vi "HW_Poll_Tracker_2.0.4+.vi"(8 "error in":errorcluster, 11 "VISA resource name in":refnum<visa-resource-name>="ASRL3::INSTR") -> (0 "error out":errorcluster, 1 "Read buffer":string, 2 "Parameters output":T1, 3 "VISA resource name out":refnum<visa-resource-name>, 4 "Sync mode status":string, 5 "Sensor board size":string)   [LabVIEW 2016]
panel:
  out "Sync mode index":i32
  out "Sensor board index":i32
  out "Sensors response":string
  out "Port data status":i32
  out "Port data status index":i32
  out "FPS status":i32
  out "Poll records":u32
  out "FPS target index":i32
  out "Matrix mode status":string
  out "Matrix mode index":i32
  out "Coordinate mode status":string
  out "Coordinate mode index":i32
  out "Binary mode status":string
  out "Binary mode index":i32
  out "Array of tokens":string[](array[string])
  out "token index":i32
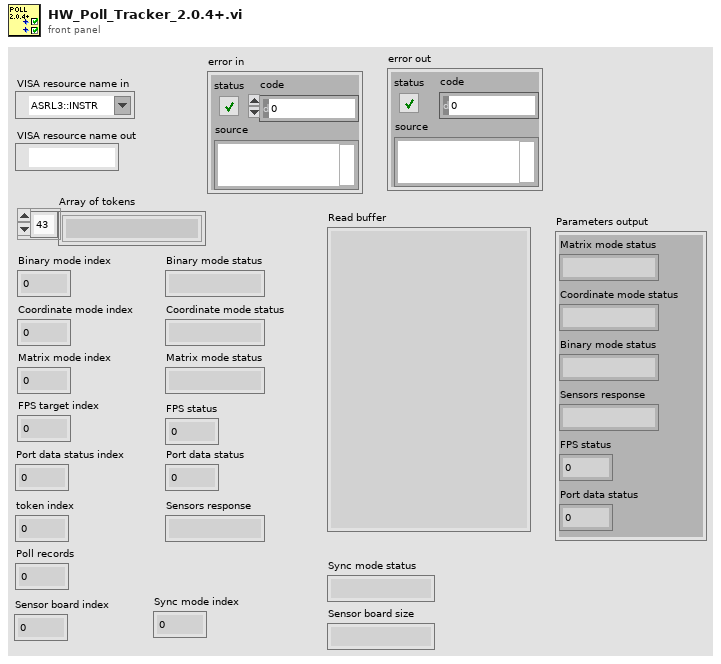
[diagram p1: front panel]
types:
  T1 = cluster{"Matrix mode status":string, "Coordinate mode status":string, "Binary mode status":string, "Sensors response":string, "FPS status":i32, "Port data status":i32}
  T2 = cluster{"token string":string, "token string":string, "token string":string, "trimmed string":string, i32, i32}
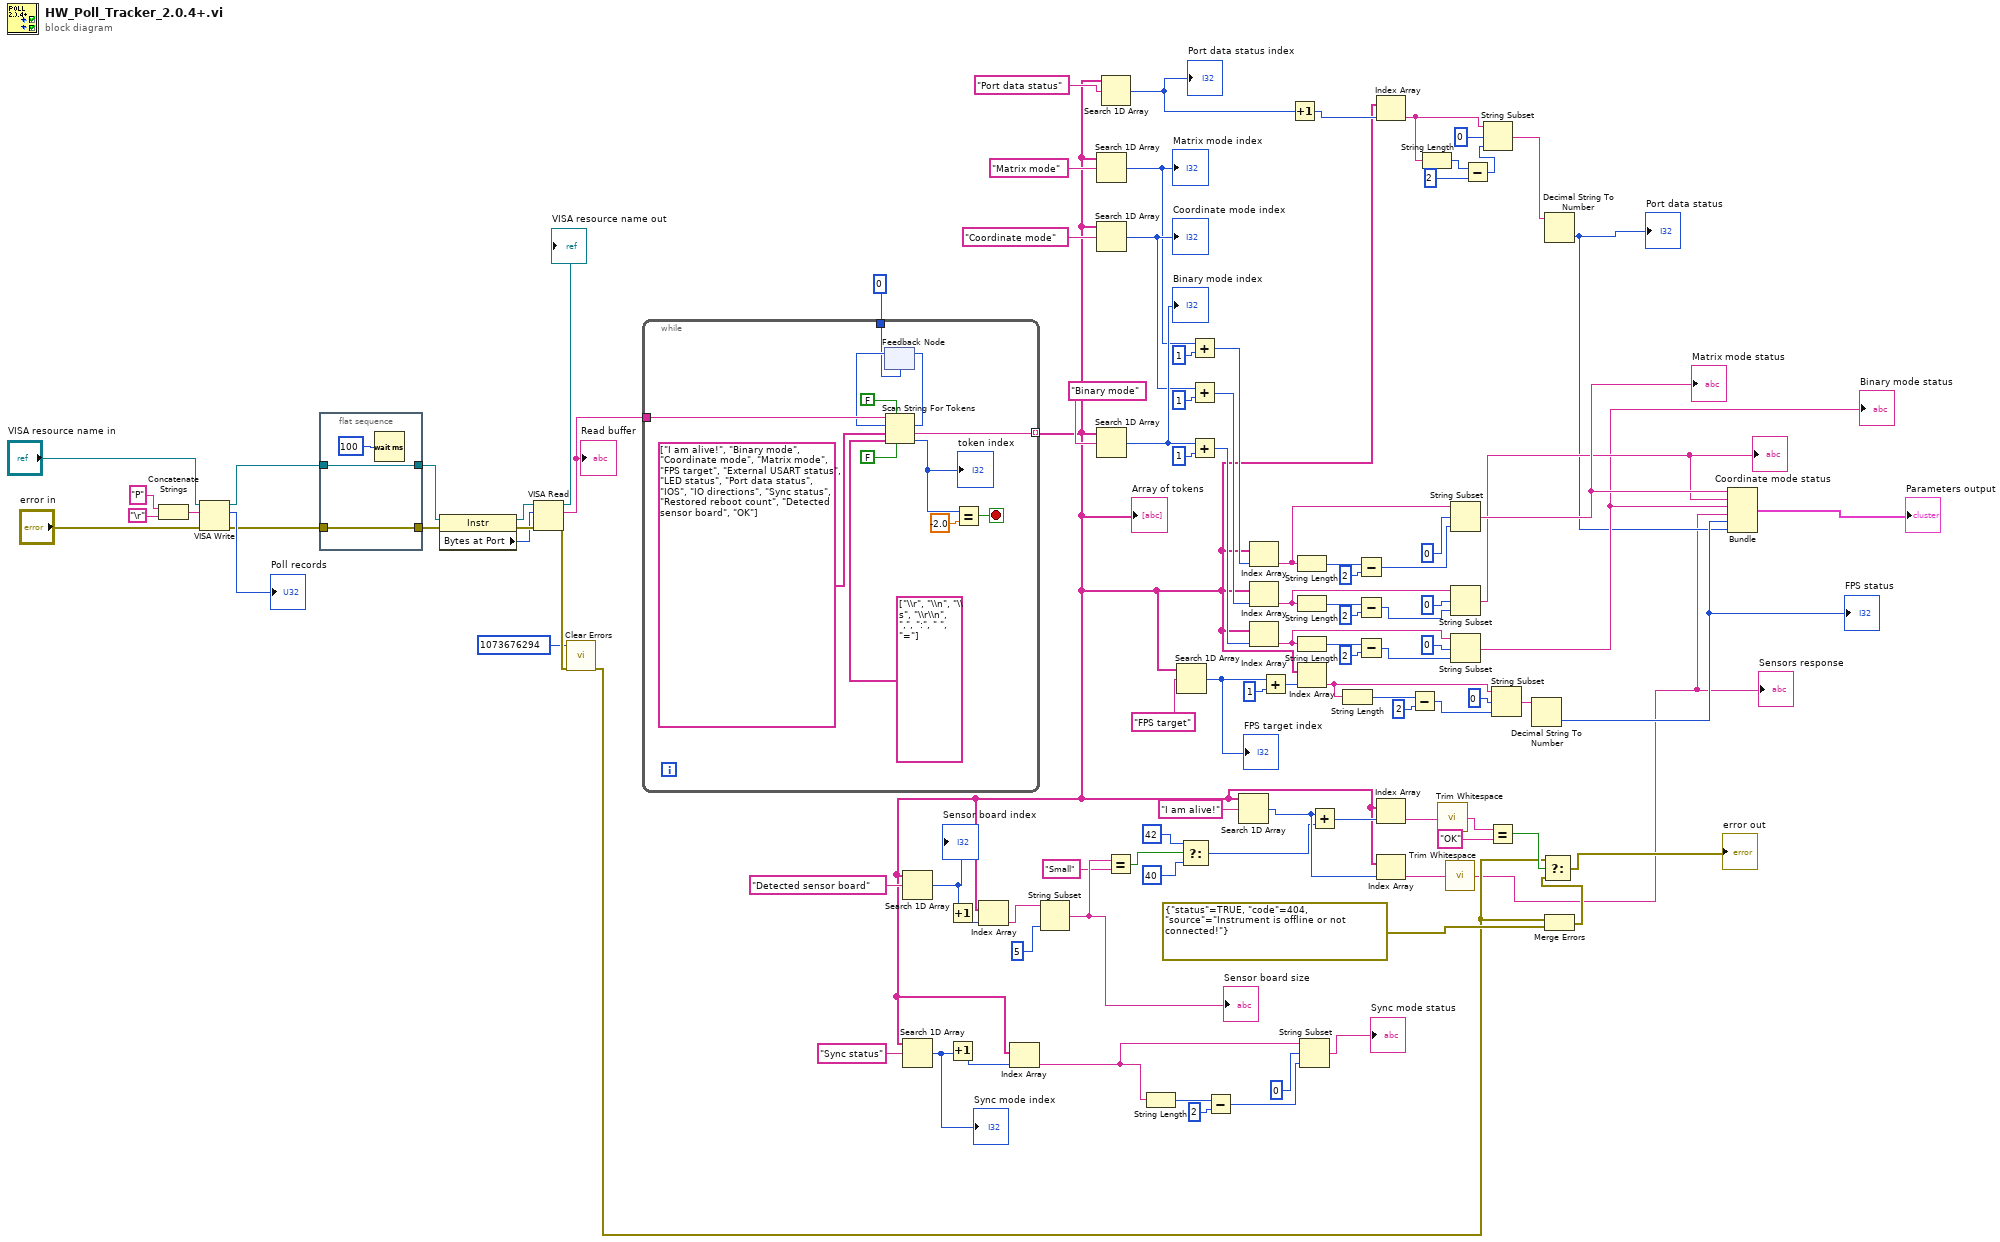
[diagram p0: block diagram]
diagram:
  n1 = Concatenate Strings("P" ("write buffer"), "\r") -> (w102:string)
  n2 = VISA Write(VISA resource name="VISA resource name in", write buffer=w102, error in (no error)="error in") -> (VISA resource name out=w77:refnum<visa-resource-name>, return count=→"Poll records":u32, error out=w75:errorcluster)
  n3 = flat-sequence {
    tunnel: [w106] -> w78
    tunnel: w77 -> [w106]
    tunnel: [w105] -> w76
    tunnel: w75 -> [w105]
    frame #0 {
      n4 = Wait (ms)(milliseconds to wait=u32 100) -> ()  [unwired: 1 out]
    }
  }
  n5 = property class="Instr"(reference=w78, error in=w76) -> (reference out=w100:refnum<visa-resource-name>, error out=w99:errorcluster, "Bytes at Port"=w98:u32)
  n6 = VISA Read(VISA resource name=w100, byte count=w98, error in (no error)=w99) -> (VISA resource name out=→"VISA resource name out":refnum<visa-resource-name>, read buffer=w97:string, error out=w35:errorcluster)  [unwired: 1 out]
  "Read buffer" <- w97
  n7 = call <vilib>:"Clear Errors.vi"("error in (no error)"=w35, "specific error code to clear (0: all)"=1073676294) -> ("error out"=w34:errorcluster)  [unwired: 4 in, 1 out]
  n8 = while {
    tunnel: w97 -> [w119]
    tunnel: [w109] -> w17 mode=indexing
    tunnel: 0 ("offset past token") -> [w108]
    stop <- w115 stop-if-true
    n9 = feedback #1(w108) -> (w116:i32)
    n10 = Scan String For Tokens(4:FALSE ("use cached delim/oper data? (F)"), 5:FALSE ("allow empty tokens? (F)"), 6:string[] ["\\r", "\\n", "\\s", "\\r\\n", ",", ":", " ", "="] ("delimiters"), 7:string[] ["I am alive!", "Binary mode", "Coordinate mode", "Matrix mode", "FPS target", "External USART status", "LED status", "Port data status", "IOS", "IO directions", "Sync status", "Restored reboot count", "Detected sensor board", "OK"] ("Tokens"), 8:w116, 9:w119) -> (0:w113:i32, 1:w109:string, 2:w117:i32)  [unwired: 1 out]
    "token index" <- w113
    n11 = feedback-in #1(w117) -> ()
    n12 = Equal?(x=w113, y=-2.0) -> (x = y?=w115:bool)
  }
  "Array of tokens" <- w17
  n13 = Search 1D Array(1D array=w17, element="Detected sensor board") -> (index of element=w23:i32)  [unwired: 1 in]
  "Sensor board index" <- w23
  n14 = Search 1D Array(1D array=w17, element="Sync status") -> (index of element=w10:i32)  [unwired: 1 in]
  "Sync mode index" <- w10
  n15 = Increment(x=w23) -> (x+1=w22:i32)
  n16 = Increment(x=w10) -> (x+1=w18:i32)
  n17 = Index Array(array=w17, index=w22) -> (element=w21:string)
  n18 = Index Array(array=w17, index=w18) -> (element=w11:string)
  n19 = String Subset(string=w21, length (rest)=5 ("length (rest)")) -> (substring=w6:string)  [unwired: 1 in]
  "Sensor board size" <- w6
  n20 = Search 1D Array(1D array=w17, element="Matrix mode") -> (index of element=w86:i32)  [unwired: 1 in]
  "Matrix mode index" <- w86
  n21 = Search 1D Array(1D array=w17, element="Coordinate mode") -> (index of element=w90:i32)  [unwired: 1 in]
  "Coordinate mode index" <- w90
  n22 = Search 1D Array(1D array=w17, element="Binary mode") -> (index of element=w94:i32)  [unwired: 1 in]
  "Binary mode index" <- w94
  n23 = Search 1D Array(1D array=w17, element="Port data status") -> (index of element=w51:i32)  [unwired: 1 in]
  "Port data status index" <- w51
  n24 = Equal?(x=w6, y="Small") -> (x = y?=w4:bool)
  n25 = String Length(string=w11) -> (length=w14:i32)
  n26 = Search 1D Array(1D array=w17, element="FPS target") -> (index of element=w82:i32)  [unwired: 1 in]
  "FPS target index" <- w82
  n27 = Select(t=42, s=w4, f=40 ("y")) -> (s? t:f=w2:i32)
  n28 = Add(x=w86, y=1) -> (x+y=w87:i32)
  n29 = Add(x=w90, y=1) -> (x+y=w91:i32)
  n30 = Add(x=w94, y=1) -> (x+y=w95:i32)
  n31 = Subtract(x=w14, y=2) -> (x-y=w16:i32)
  n32 = Search 1D Array(1D array=w17, element="I am alive!") -> (index of element=w9:i32)  [unwired: 1 in]
  n33 = Index Array(array=w17, index=w87) -> (element=w55:string)
  n34 = Index Array(array=w17, index=w91) -> (element=w53:string)
  n35 = Index Array(array=w17, index=w95) -> (element=w72:string)
  n36 = Add(x=w82, y=1) -> (x+y=w83:i32)
  n37 = Increment(x=w51) -> (x+1=w50:i32)
  n38 = String Length(string=w55) -> (length=w67:i32)
  n39 = String Length(string=w53) -> (length=w58:i32)
  n40 = String Length(string=w72) -> (length=w71:i32)
  n41 = Index Array(array=w17, index=w83) -> (element=w54:string)
  n42 = String Subset(string=w11, offset (0)=0, length (rest)=w16) -> (substring=→"Sync mode status":string)
  n43 = Add(x=w9, y=w2) -> (x+y=w32:i32)
  n44 = String Length(string=w54) -> (length=w63:i32)
  n45 = Subtract(x=w67, y=2) -> (x-y=w65:i32)
  n46 = Subtract(x=w58, y=2) -> (x-y=w56:i32)
  n47 = Subtract(x=w71, y=2) -> (x-y=w69:i32)
  n48 = Index Array(array=w17, index=w50) -> (element=w49:string)
  n49 = Index Array(array=w17, index=w32) -> (element=w42:string)
  n50 = Index Array(array=w17, index=w9) -> (element=w8:string)
  n51 = Subtract(x=w63, y=2) -> (x-y=w61:i32)
  n52 = String Length(string=w49) -> (length=w48:i32)
  n53 = call <vilib>:"Trim Whitespace.vi"("string"=w42) -> ("trimmed string"=w41:string)  [unwired: 1 in]
  n54 = call <vilib>:"Trim Whitespace.vi"("string"=w8) -> ("trimmed string"=w7:string)  [unwired: 1 in]
  "Sensors response" <- w7
  n55 = String Subset(string=w55, offset (0)=0, length (rest)=w65) -> (substring=w30:string)
  "Matrix mode status" <- w30
  n56 = String Subset(string=w53, offset (0)=0, length (rest)=w56) -> (substring=w29:string)
  "Coordinate mode status" <- w29
  n57 = String Subset(string=w72, offset (0)=0, length (rest)=w69) -> (substring=w28:string)
  "Binary mode status" <- w28
  n58 = Subtract(x=w48, y=2) -> (x-y=w46:i32)
  n59 = String Subset(string=w49, offset (0)=0, length (rest)=w46) -> (substring=w44:string)
  n60 = Equal?(x=w41, y="OK") -> (x = y?=w39:bool)
  n61 = String Subset(string=w54, offset (0)=0, length (rest)=w61) -> (substring=w60:string)
  n62 = Decimal String To Number(string=w60) -> (number=w27:i32)  [unwired: 2 in, 1 out]
  "FPS status" <- w27
  n63 = Decimal String To Number(string=w44) -> (number=w26:i32)  [unwired: 2 in, 1 out]
  "Port data status" <- w26
  n64 = Merge Errors(w34, errorcluster {"status"=TRUE, "code"=404, "source"="Instrument is offline or not connected!"} ("error in")) -> (w37:errorcluster)
  n65 = Select(t=w34, s=w39, f=w37) -> (s? t:f=→"error out":errorcluster)
  n66 = Bundle("token string"=w30, "token string"=w29, "token string"=w28, "trimmed string"=w7, w27, w26) -> (→"Parameters output":T2)  [unwired: 1 in]
